vi "parse.printPrice.vi"(7 "prices":cluster{"price":dbl, "type":string}[](array[cluster])) -> (3 "price":sgl)   [LabVIEW 2024]
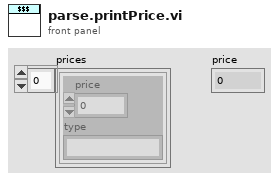
[diagram p1: front panel]
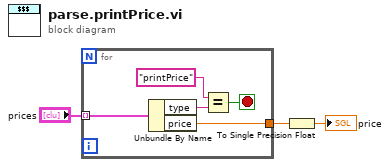
[diagram p0: block diagram]
diagram:
  n1 = for {
    tunnel: "prices" -> [w8] mode=indexing
    tunnel: [w7] -> w2
    stop <- w4 stop-if-true
    n2 = Unbundle By Name(w8) -> ("type"=w6:string, "price"=w7:dbl)
    n3 = Equal?(x="printPrice", y=w6) -> (x = y?=w4:bool)
  }
  n4 = To Single Precision Float(number=w2) -> (single precision float=→"price":sgl)
